vi "Position Conversion.vi"(0 "Child Hwnd":u32, 5 "Parent Position":T2, 11 "error in (no error)":errorcluster) -> (4 "Child Position":T1, 15 "error out":errorcluster)   [LabVIEW 2016, in "LV MDI.lvclass"]
uses:
  LV MDI.lvclass
  TypeDefs/Offset Rect.ctl
  TypeDefs/Set Position.ctl
  user32.dll
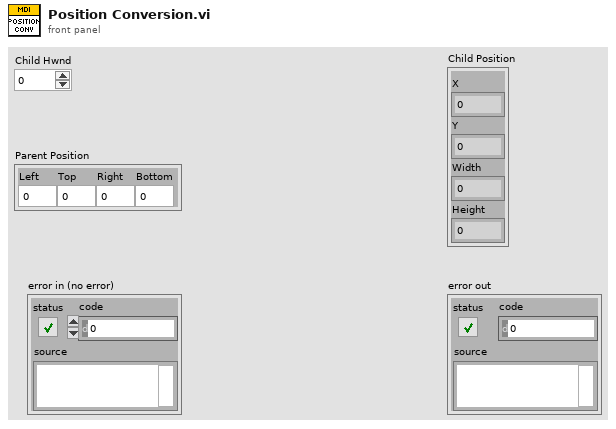
[diagram p1: front panel]
types:
  T1 = typedef "LV MDI.lvclass/Set Position.ctl" = cluster{"X":i32, "Y":i32, "Width":i32, "Height":i32}
  T2 = typedef "LV MDI.lvclass/Offset Rect.ctl" = cluster{"Left":i32, "Top":i32, "Right":i32, "Bottom":i32}
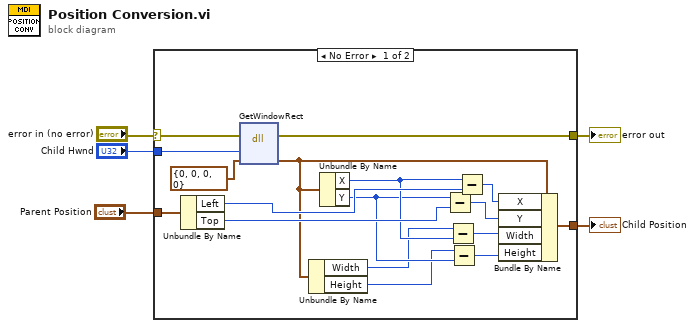
[diagram p0: block diagram]
diagram:
  n1 = case shown="No Error" "error in (no error)" {
    selector: "error in (no error)" -> [w15 w23]
    tunnel: "Parent Position" -> [w20 _]
    tunnel: [w19 _] -> w4
    tunnel: "Child Hwnd" -> [w17 _]
    tunnel: [w16 w23] -> w2
    frame No Error {
      n2 = Unbundle By Name(w20) -> ("Left"=w21:i32, "Top"=w22:i32)
      n3 = dll-call lib="user32.dll" fn="GetWindowRect"(error in=w15, "Hwnd"=w17, "lpRect"=T1 {"X"=0, "Y"=0, "Width"=0, "Height"=0} ("Position")) -> (error out=w16:errorcluster, "lpRect"=w8:T1)  [unwired: 4 in, 1 out]
      n4 = Unbundle By Name(w8) -> ("Width"=w7:i32, "Height"=w6:i32)
      n5 = Unbundle By Name(w8) -> ("X"=w12:i32, "Y"=w9:i32)
      n6 = Subtract(x=w9, y=w22) -> (x-y=w11:i32)
      n7 = Subtract(x=w7, y=w12) -> (x-y=w13:i32)
      n8 = Subtract(x=w6, y=w9) -> (x-y=w10:i32)
      n9 = Subtract(x=w12, y=w21) -> (x-y=w14:i32)
      n10 = Bundle By Name(cluster=w8, "X"=w14, "Y"=w11, "Width"=w13, "Height"=w10) -> (w19:T1)
    }
    frame Error {
    }
  }
  "Child Position" <- w4
  "error out" <- w2
